vi "z_control_statemachine_FP_forv4.vi"(4 "TF-params":T2={"TF-order"=0, "Num"=[0.0, 0.0, 0.0, 0.0, 0.0, 0.0, 0.0, 0.0, 0.0], "Den"=[0.0, 0.0, 0.0, 0.0, 0.0, 0.0, 0.0, 0.0, 0.0]}, 7 "do-Dz":bool, 8 "z_axis_params":T1={"TOL"=0.3, "z_u_max"=5.0, "setpoint-scan"=0.0, "Ki-scan"=0.001, "Z_error_threshold"=0.0, "Z_settled_samples_threshold "=0, "uz_safe"=0.0, "Kiz_down"=0.001, "max_Z_settle_samples"=5000, "setpoint-up"=0.0} {"uz_safe" format="%#_13g"; "Z_error_threshold" format="%#_13g"; "TOL" format="%#_13g"}, 10 "State":u8, 11 "zerr(k)":sgl) -> (2 "zuk_Dinv":fxp<+/-,16,5>, 3 "z-u(k)":fxp<+/-,16,5>)   [LabVIEW 2017]
uses:
  controls/TF-params.ctl
  controls/z-axis-params_v4.ctl
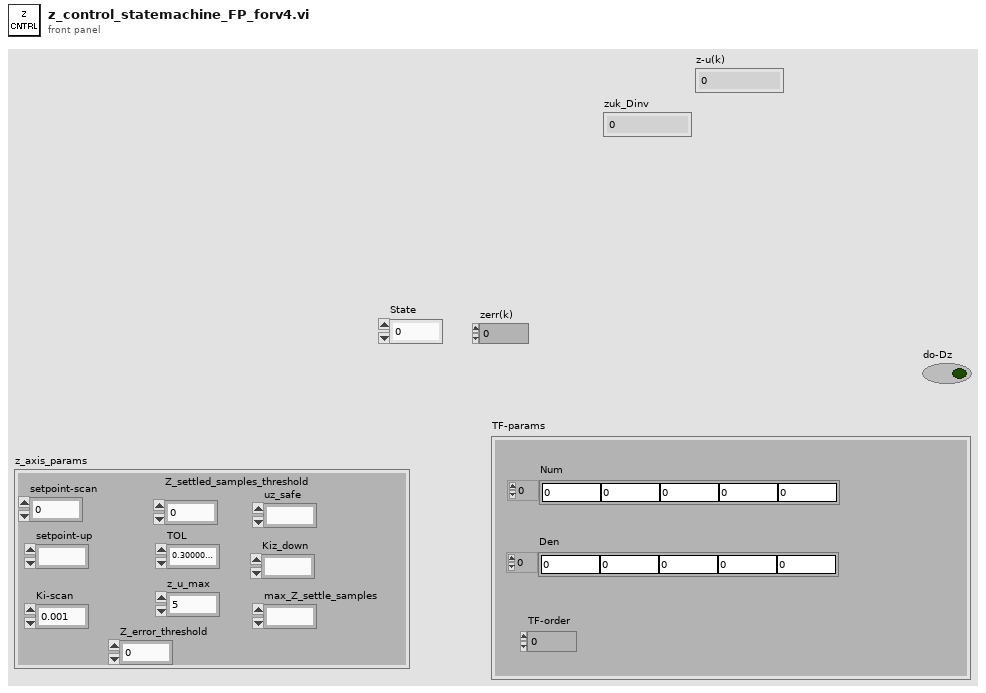
[diagram p1: front panel]
types:
  T1 = typedef "z-axis-params_v4.ctl" = cluster{"TOL":sgl, "z_u_max":sgl, "setpoint-scan":sgl, "Ki-scan":sgl, "Z_error_threshold":sgl, "Z_settled_samples_threshold ":i16, "uz_safe":fxp<+/-,16,5>, "Kiz_down":sgl, "max_Z_settle_samples":i16, "setpoint-up":sgl}
  T2 = typedef "TF-params.ctl" = cluster{"TF-order":i16, "Num":sgl[], "Den":sgl[]}
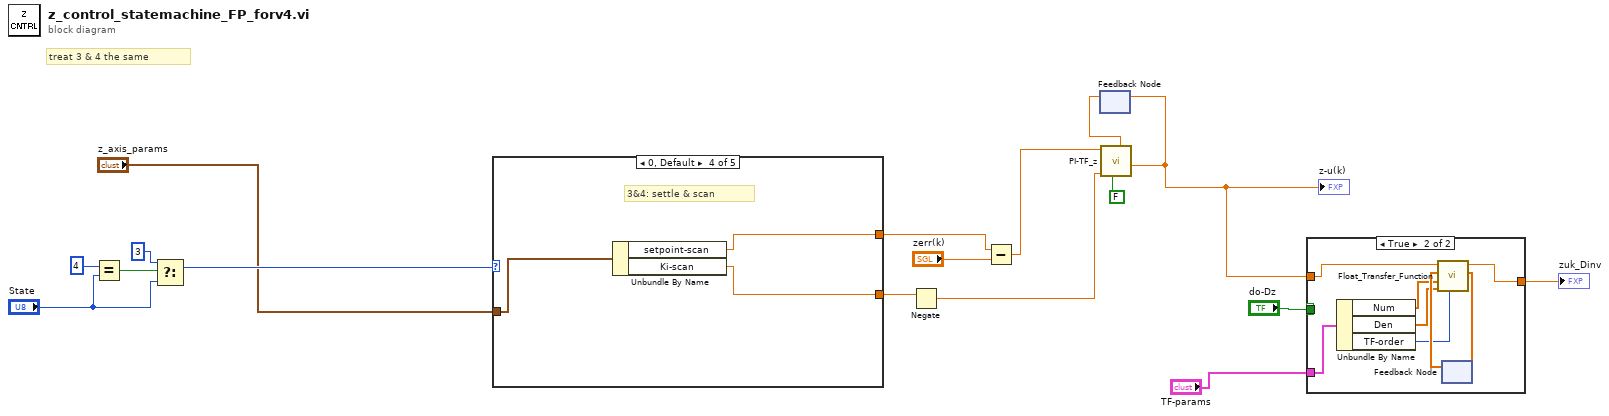
[diagram p0: block diagram]
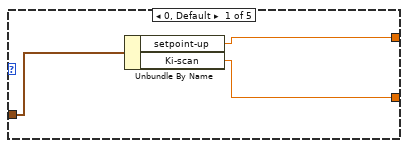
[diagram p3: hidden frame]
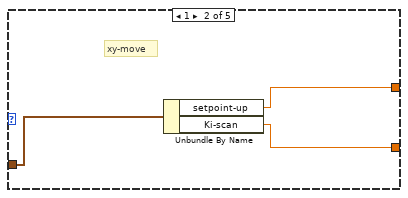
[diagram p4: hidden frame]
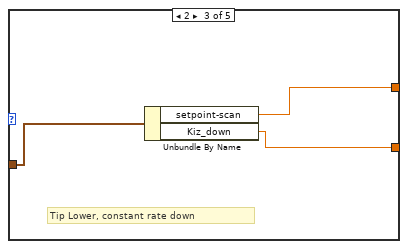
[diagram p5: hidden frame]
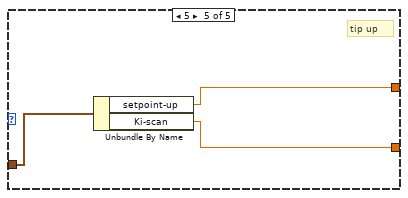
[diagram p6: hidden frame]
diagram:
  # "treat 3 & 4 the same"
  n1 = Equal?(x=i8 4 ("y"), y="State") -> (x = y?=w16:bool)
  n2 = Select(t=i8 3 ("y"), s=w16, f="State") -> (s? t:f=w14:u8)
  n3 = case shown="0, Default" w14 {
    tunnel: "z_axis_params" -> [w20 w23 w26 w29 w32]
    tunnel: [w18 w21 w24 w27 w30] -> w4
    tunnel: [w19 w22 w25 w28 w31] -> w1
    frame 0, Default {
      n4 = Unbundle By Name(w20) -> ("setpoint-up"=w19:sgl, "Ki-scan"=w18:sgl)
    }
    frame 1 {
      # "xy-move"
      n5 = Unbundle By Name(w23) -> ("setpoint-up"=w22:sgl, "Ki-scan"=w21:sgl)
    }
    frame 2 {
      # "Tip Lower, constant rate down"
      n6 = Unbundle By Name(w26) -> ("setpoint-scan"=w25:sgl, "Kiz_down"=w24:sgl)
    }
    frame 3 {
      # "3&4: settle & scan"
      n7 = Unbundle By Name(w29) -> ("setpoint-scan"=w28:sgl, "Ki-scan"=w27:sgl)
    }
    frame 5 {
      # "tip up"
      n8 = Unbundle By Name(w32) -> ("setpoint-up"=w31:sgl, "Ki-scan"=w30:sgl)
    }
  }
  n9 = Negate(x=w4) -> (-x=w3:sgl)
  n10 = Subtract(x=w1, y="zerr(k)") -> (x-y=w2:sgl)
  n11 = feedback #1() -> (w7:sgl)  [unwired: 1 in]
  n12 = call "PI-TF_z.vi"("u(k-1)"=w7, "reset"=FALSE, "Ki"=w3, "e(k)"=w2) -> ("u(k)"=w5:sgl)  [unwired: 7 in]
  "z-u(k)" <- w5
  n13 = feedback-in #1(w5) -> ()
  n14 = case shown="False" "do-Dz" {
    tunnel: "do-Dz" -> [_ _]
    tunnel: w5 -> [w33 w36]
    tunnel: [w33 w37] -> w9
    tunnel: "TF-params" -> [_ w35]
    frame False {
    }
    frame True {
      n15 = Unbundle By Name(w35) -> ("Num"=w39:sgl[], "Den"=w38:sgl[], "TF-order"=w34:i16)
      n16 = feedback #2() -> (w40:sgl[])  [unwired: 1 in]
      n17 = call "Float_Transfer_Function.vi"("TF Order"=w34, "Den"=w38, "Num"=w39, "State In"=w40, "Input"=w36) -> ("State Out"=w41:sgl[], "Output"=w37:sgl)  [unwired: 4 in]
      n18 = feedback-in #2(w41) -> ()
    }
  }
  "zuk_Dinv" <- w9
